vi "cv_05_01.vi"() -> ()   [LabVIEW 2013]
panel:
  out "Small Cluster":cluster{"Boolean 1":bool, "Slide Value":dbl}
  out "Boolean":bool
  out "Numeric":dbl
  in  "stop":bool
  out "Modified Cluster":T1 {"Slide" scale=0.0..10.0}
  in  "Cluster":T1 {"Slide" scale=0.0..10.0}
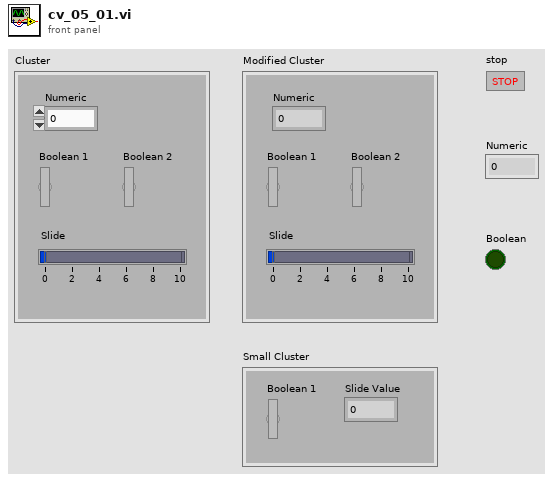
[diagram p1: front panel]
types:
  T1 = cluster{"Numeric":dbl, "Boolean 1":bool, "Boolean 2":bool, "Slide":dbl}
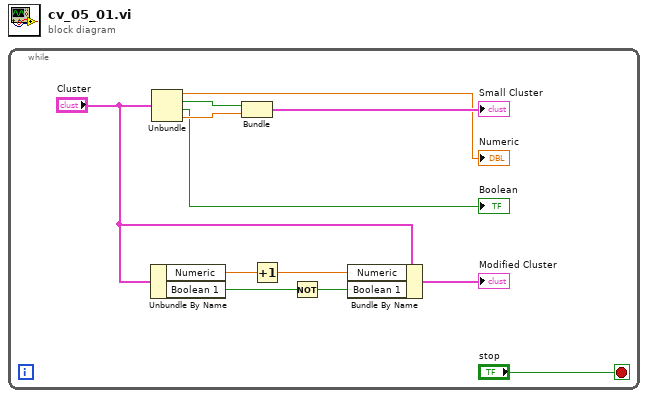
[diagram p0: block diagram]
diagram:
  n1 = while {
    stop <- "stop" stop-if-true
    n2 = Unbundle By Name("Cluster") -> ("Numeric"=w5:dbl, "Boolean 1"=w3:bool)
    n3 = Unbundle("Cluster") -> ("Numeric"=→"Numeric":dbl, "Boolean 1"=w11:bool, "Boolean 2"=→"Boolean":bool, "Slide"=w10:dbl)
    n4 = Bundle("Boolean 1"=w11, "Slide"=w10) -> (→"Small Cluster":cluster{"Boolean 1":bool, "Slide":dbl})  [unwired: 1 in]
    n5 = Increment(x=w5) -> (x+1=w4:dbl)
    n6 = Not(x=w3) -> (.not. x?=w2:bool)
    n7 = Bundle By Name(cluster="Cluster", "Numeric"=w4, "Boolean 1"=w2) -> (→"Modified Cluster":T1)
  }
